vi "ToMatlabParam.vi"(4 "Base Object Path":string, 6 "Add the container name (f)":bool, 11 "Value":variant) -> (3 "Matlab Param Data":T1[](array[typedef]))   [LabVIEW 2017]
uses:
  Types/MatlabDataBundle.ctl
  Types/MatlabDataType.ctl
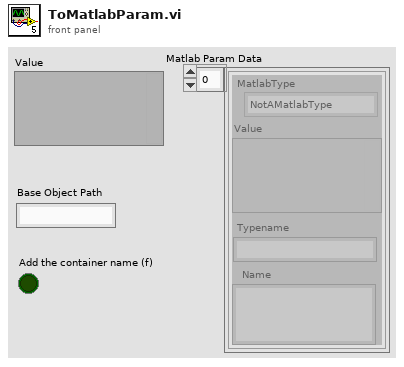
[diagram p1: front panel]
types:
  T1 = typedef "MatlabDataBundle.ctl" = cluster{"MatlabType":T2, "Value":variant, "Name":string, "Typename":string}
  T2 = typedef "MatlabDataType.ctl" = enum16{"NotAMatlabType", "Real", "Complex", "String", "Boolean"}
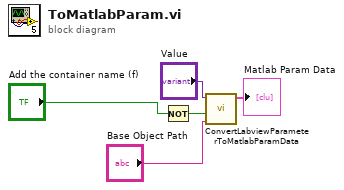
[diagram p0: block diagram]
diagram:
  n1 = Not(x="Add the container name (f)") -> (.not. x?=w1:bool)
  n2 = call "ConvertLabviewParameterToMatlabParamData.vi"("BaseName"="Base Object Path", "IgnoreContainerName"=w1, "Value"="Value") -> ("Matlab Param Data"=→"Matlab Param Data":T1[])  [unwired: 8 in]
